vi "FGV Datenmanagment.vi"(11 "error in (no error)":errorcluster caption="Fehler (Eingang, kein Fehler)", 13 "Aktion":T3=enum."lesen") -> (2 "Aktuelle Messwerte":sgl[](array[numeric]), 3 "Ergebnistabelle":string[][](array[string]), 4 "Daten":T1 {"Höchster Peak" format="%#_5g"; "T10 Grenzwert" format="%#_5g"; "FallTime gemittelt" format="%#_5g"; "T90 Grenzwert" format="%#_5g"; "RiseTime gemittelt" format="%#_5g"}, 6 "T90 Signalverlauf":waveform(sgl) caption="Waveform", 8 "Peak im Bereich":bool, 10 "Aktueller Wert":sgl, 14 "Start":timestamp, 15 "error out":errorcluster caption="Fehler (Ausgang)")   [LabVIEW 2020, in "EPA 1065.lvlib" / "T90 Test 1065-308.lvlib"]
uses:
  T90 Test 1065-308.lvlib
  Aktion FGV Datenmanagment.ctl
  Datencluster.ctl
  Visualisierungs Elemente/Zahlen-Eingabefeld.ctl
  Aktion FGV T90.ctl
  Messdaten/Aktionen FGV Messdaten.ctl
  <vilib>/Analysis/baseanly.llb/Mean (DBL).vi
  Messdaten/Messdaten.lvlib
  <vilib>/Analysis/NI_AALBase.lvlib
panel:
  out "Umschaltzeitpunkt":timestamp[](array[timestamp])
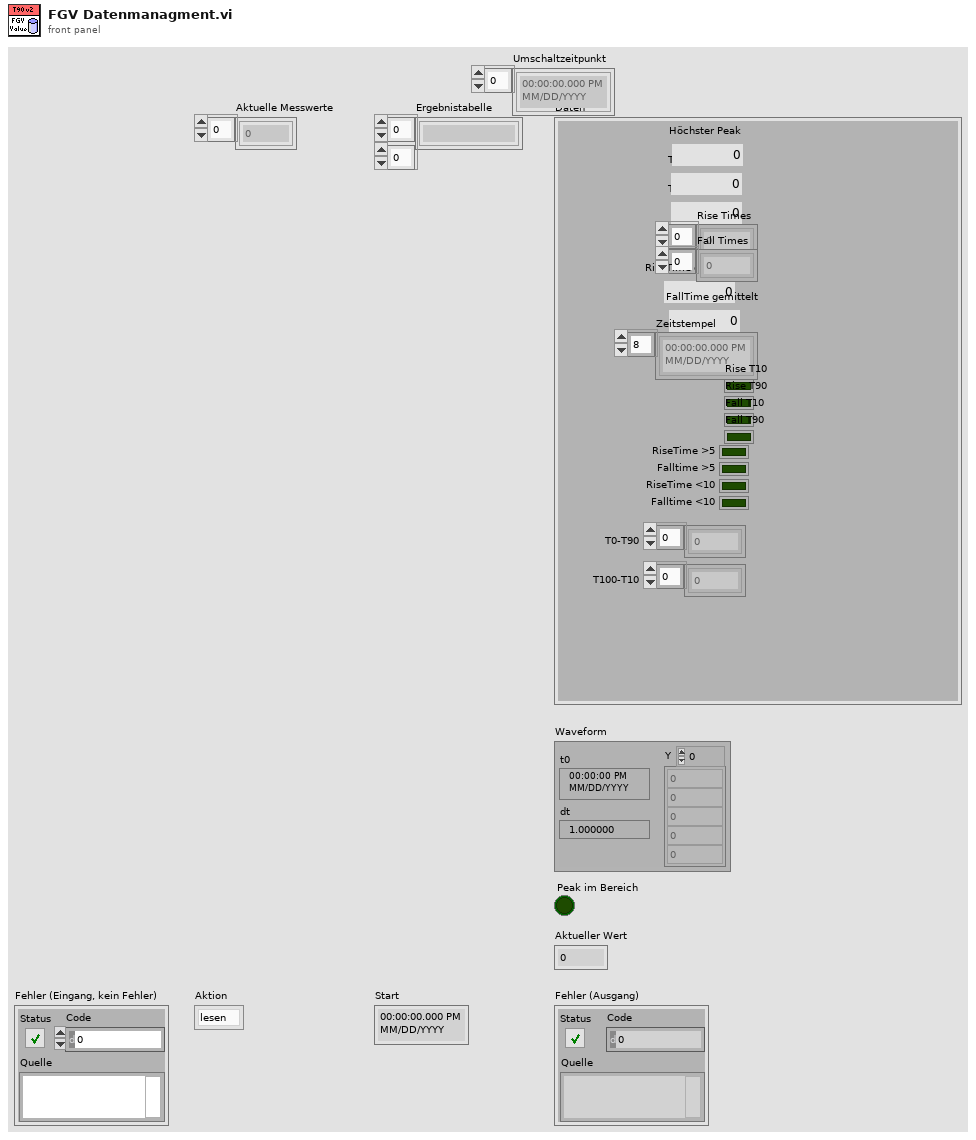
[diagram p1: front panel]
types:
  T1 = typedef "EPA 1065.lvlib/T90 Test 1065-308.lvlib/Datencluster.ctl" = cluster{"Höchster Peak":T2, "T10 Grenzwert":T2, "T90 Grenzwert":T2, "Rise Times":dbl[], "Fall Times":dbl[], "RiseTime gemittelt":T2, "FallTime gemittelt":T2, "Zeitstempel":timestamp[], "Rise T10":bool, "Rise T90":bool, "Fall T10":bool, "Fall T90":bool, "RiseTime >5":bool, "Falltime >5":bool, "RiseTime <10":bool, "Falltime <10":bool, "T0-T90":dbl[], "T100-T10":dbl[]}
  T2 = typedef "Zahlen-Eingabefeld.ctl" = sgl
  T3 = typedef "EPA 1065.lvlib/T90 Test 1065-308.lvlib/Aktion FGV Datenmanagment.ctl" = enum16{"init", "lesen", "Istwerte schreiben", "höchsten Peak setzen", "Auswerten", "Grenzen setzen", "Sollwert ändern", "Rise T10", "Rise T90", "Fall T90", "Fall T10", "Bit löschen", "Umschaltzeitpunkt"}
  T4 = typedef "EPA 1065.lvlib/T90 Test 1065-308.lvlib/Aktion FGV T90.ctl" = enum16{"lesen", "Konfig Daten", "speichern", "laden", "T90 aktiv", "T90 inaktiv", "Ext. Ventil aktivieren", "Ext. Ventil deaktivieren", "N2 spülen aktiv", "N2 spülen inaktiv", "Ergebnis Textfile"}
  T5 = typedef "Messdaten.lvlib/Aktionen FGV Messdaten.ctl" = enum16{"lesen", "schreiben", "löschen", "Mittelwerte", "Komponente"}
  T6 = typedef "EPA 1065.lvlib/T90 Test 1065-308.lvlib/T90 Konfig Daten.ctl" = cluster{"Bearbeiter:":string, "Komponente:":u16, "Gasflaschen Nr.:":string, "Accuracy":dbl, "Sollwert":dbl, "Modus":T7, "Abschaltzeit:":dbl, "Abweichung:":dbl, "Pfad:":path, "Textname:":string, "CG Aufschaltzeit:":dbl, "Einheit":string, "N2 Aufschaltzeit:":dbl, "Analysator":T8, "Gasflasche":T9, "Konfig Gasflasche":T10, "Frequency:":T11}
  T7 = typedef "EPA 1065.lvlib/T90 Test 1065-308.lvlib/Modus.ctl" = u16
  T8 = typedef "System Einstellungen V2.lvlib/Analysatoren.ctl" = string
  T9 = typedef "System Einstellungen V2.lvlib/Gasflasche Auswahl.ctl" = u16
  T10 = typedef "System Einstellungen V2.lvlib/Konfig Gasflasche.ctl" = bool
  T11 = typedef "EPA 1065.lvlib/T90 Test 1065-308.lvlib/Frequenz.ctl" = u16
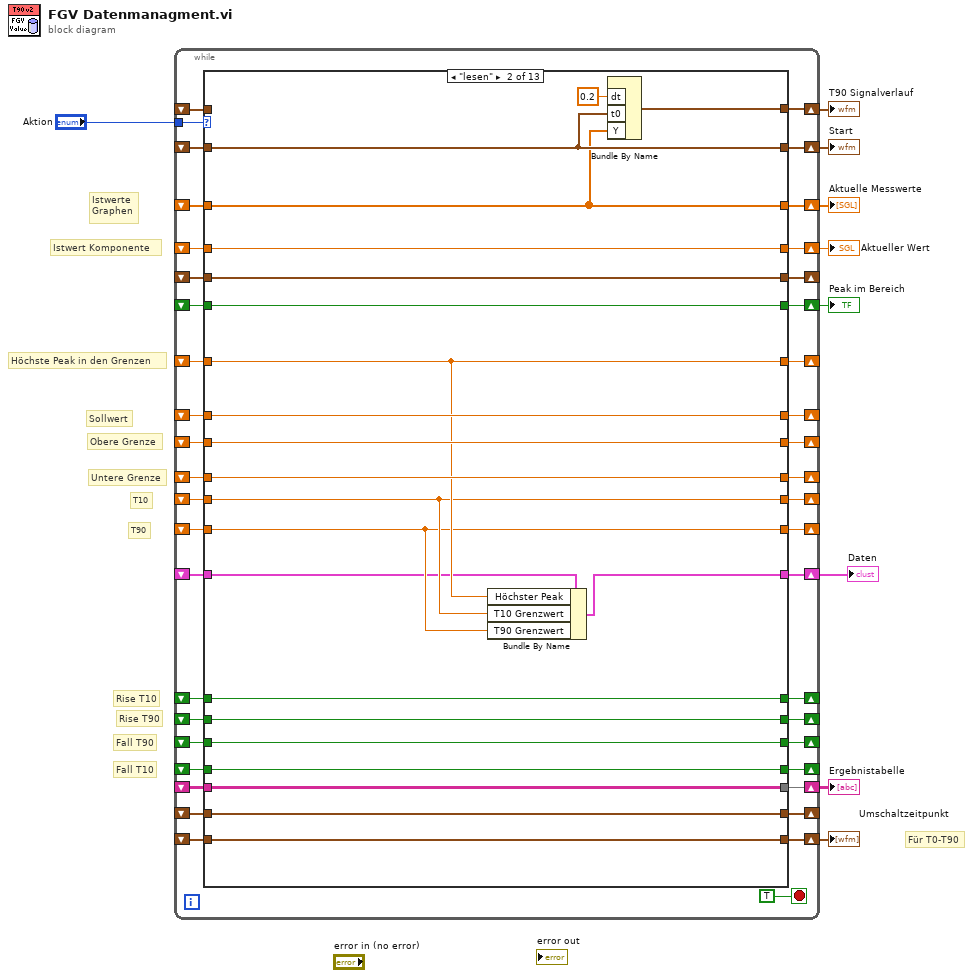
[diagram p0: block diagram]
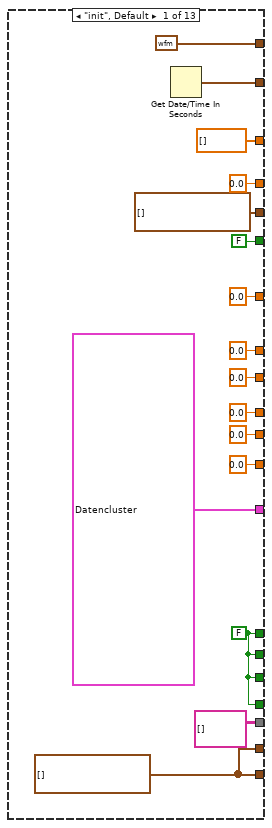
[diagram p2: hidden frame]
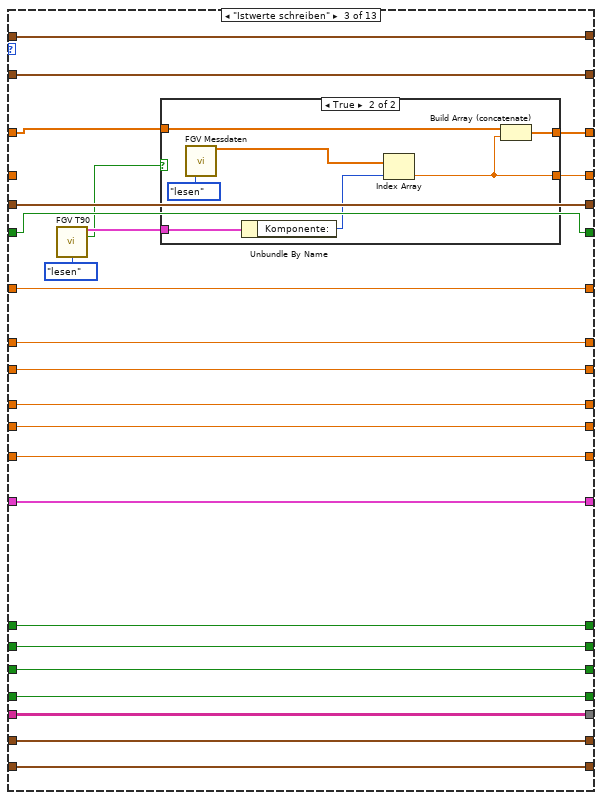
[diagram p3: hidden frame]
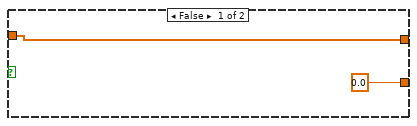
[diagram p4: hidden frame]
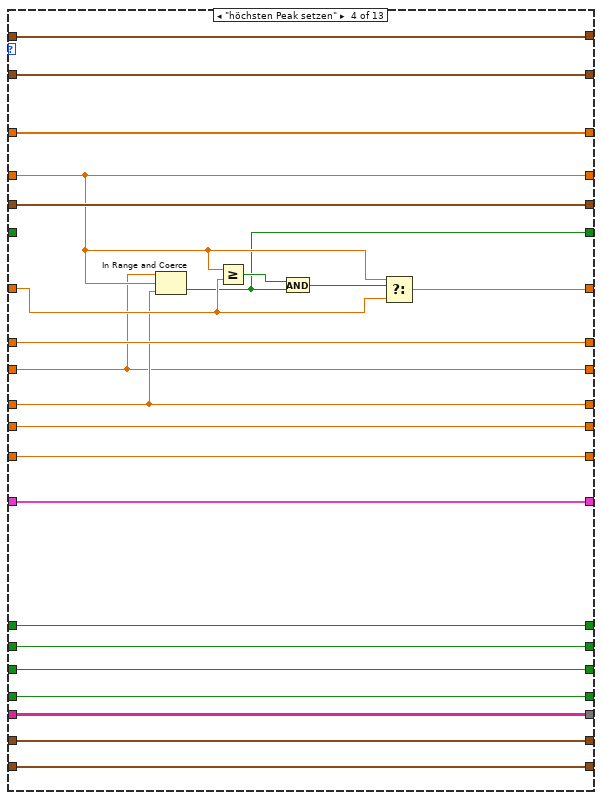
[diagram p5: hidden frame]
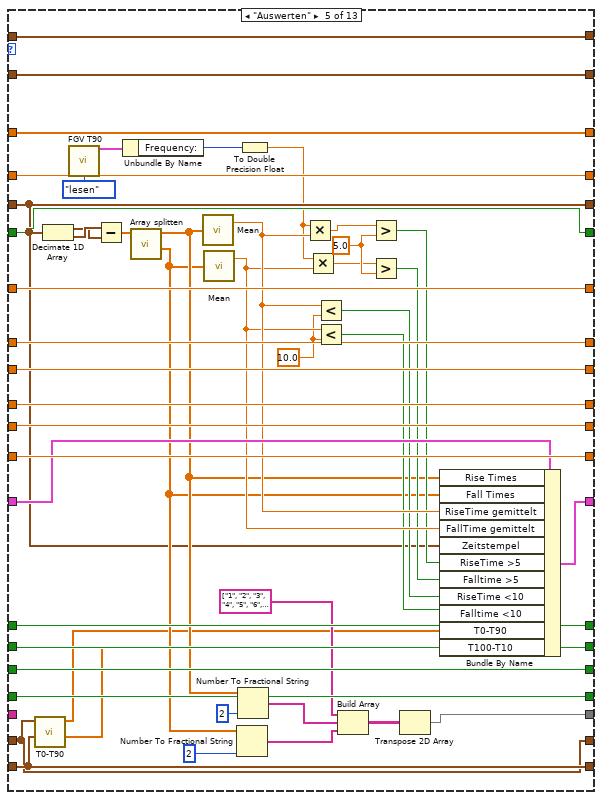
[diagram p6: hidden frame]
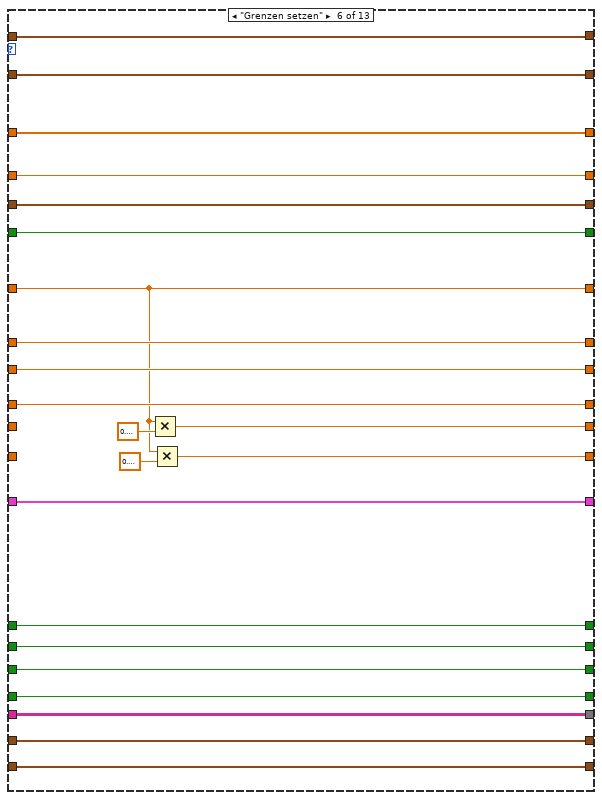
[diagram p7: hidden frame]
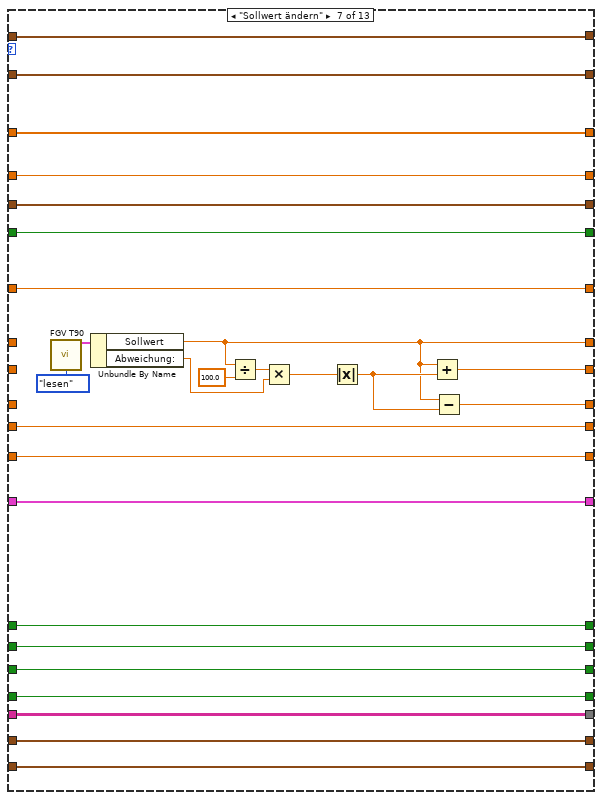
[diagram p8: hidden frame]
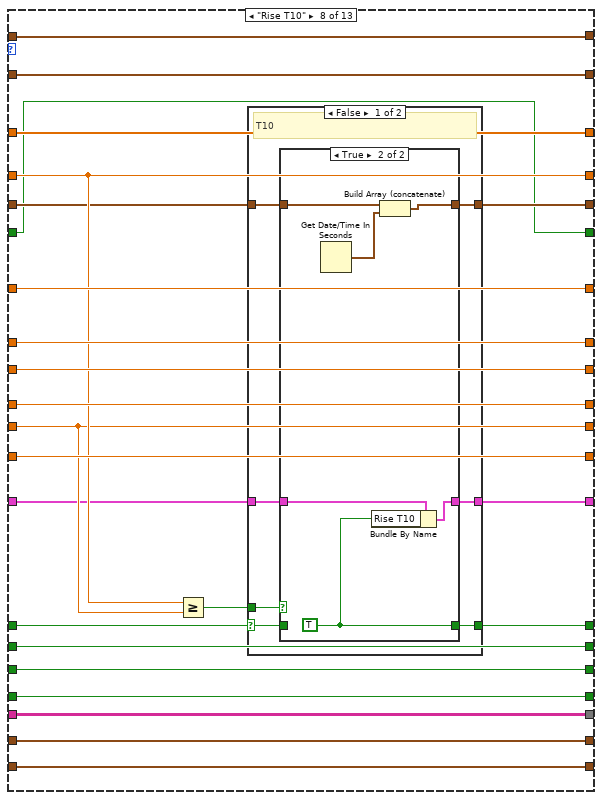
[diagram p9: hidden frame]
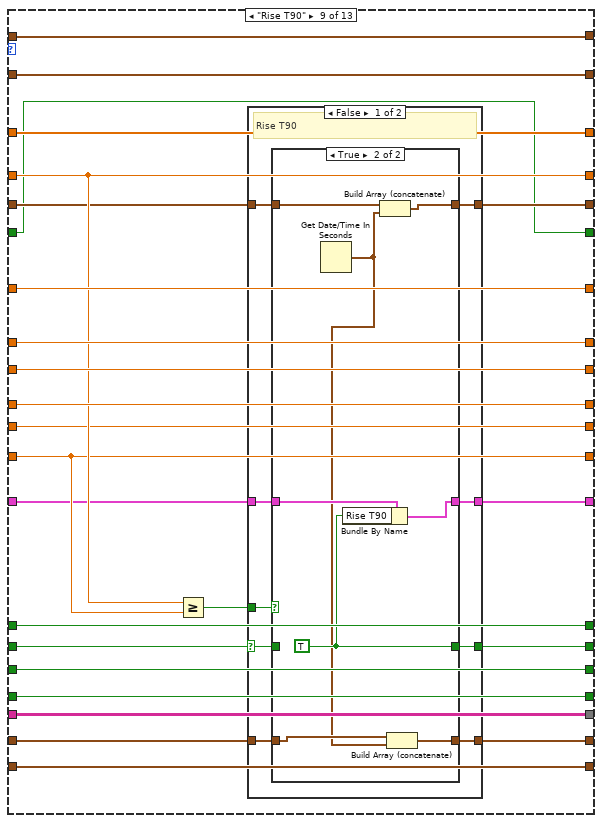
[diagram p12: hidden frame]
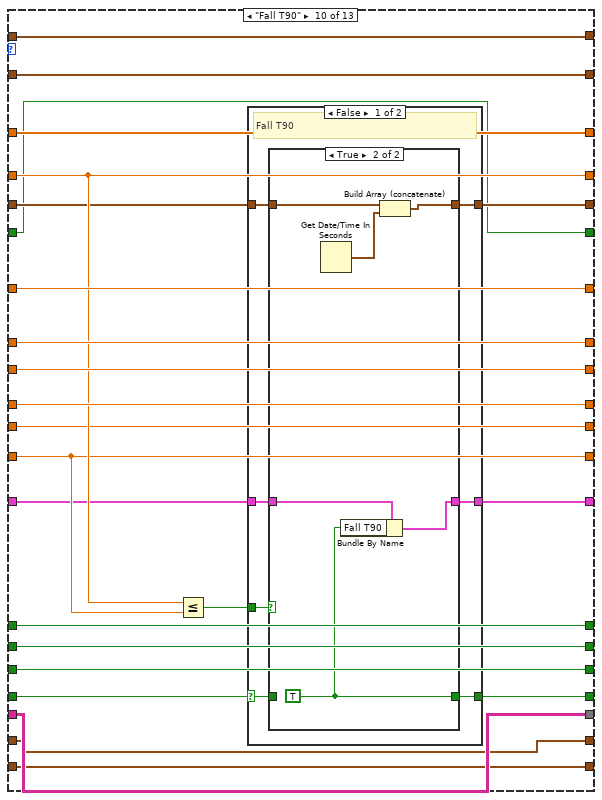
[diagram p15: hidden frame]
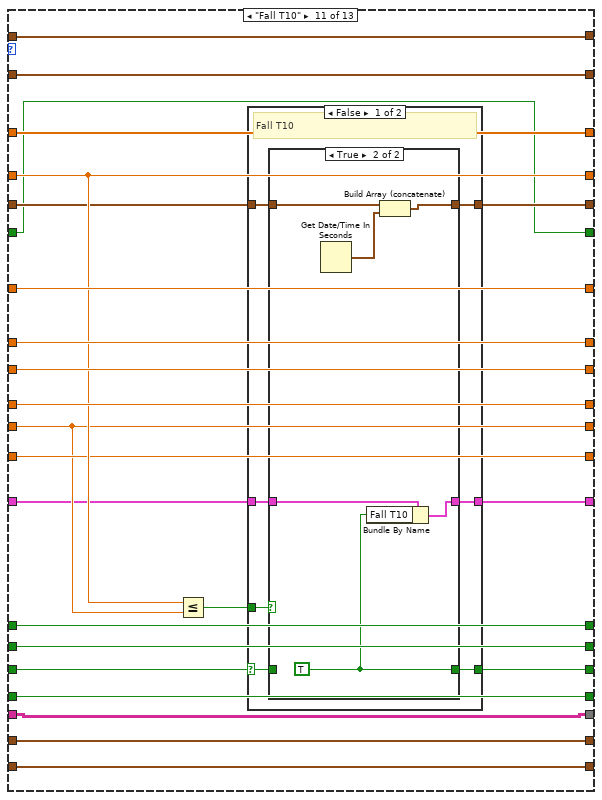
[diagram p18: hidden frame]
diagram:
  # "Für T0-T90"
  # "Fall T10"
  # "Fall T90"
  # "Rise T90"
  # "Rise T10"
  # "T90"
  # "T10"
  # "Untere Grenze"
  # "Obere Grenze"
  # "Sollwert"
  # "Höchste Peak in den Grenzen"
  # "Istwert Komponente"
  # "Istwerte\nGraphen"
  n1 = while {
    tunnel: "Aktion" -> [w50]
    shift-right: [w49] -> w1
    shift-left: _ -> [w48]
    shift-right: [w47] -> _
    shift-left: _ -> [w46]
    shift-right: [w45] -> w8
    shift-left: _ -> [w44]
    shift-right: [w43] -> _
    shift-left: _ -> [w42]
    shift-right: [w39] -> _
    shift-left: _ -> [w38]
    shift-right: [w41] -> _
    shift-left: _ -> [w37]
    shift-right: [w40] -> _
    shift-left: _ -> [w36]
    shift-right: [w35] -> _
    shift-left: _ -> [w34]
    shift-right: [w33] -> _
    shift-left: _ -> [w32]
    shift-right: [w31] -> w7
    shift-left: _ -> [w30]
    shift-right: [w28] -> _
    shift-left: _ -> [w27]
    shift-right: [w25] -> _
    shift-left: _ -> [w26]
    shift-right: [w23] -> _
    shift-left: _ -> [w24]
    shift-right: [w21] -> _
    shift-left: _ -> [w22]
    shift-right: [w20] -> w3
    shift-left: _ -> [w19]
    shift-right: [w18] -> w5
    shift-left: _ -> [w17]
    shift-right: [w16] -> w4
    shift-left: _ -> [w15]
    shift-right: [w29] -> w6
    shift-left: _ -> [w14]
    shift-right: [w13] -> w2
    shift-left: _ -> [w12]
    shift-right: [w11] -> _
    shift-left: _ -> [w10]
    stop <- TRUE stop-if-true
    n2 = case shown="\"lesen\"" w50 {
      tunnel: [sgl[] [] ("Aktuelle Messwerte") w74 w101 w145 w193 w215 w236 w266 w310 w359 w402 w436 w452] -> w49
      tunnel: w48 -> [_ w74 w100 w145 w193 w215 w236 w266 w310 w359 w402 w436 w452]
      tunnel: [timestamp[] [] w89 w113 w144 w154 w213 w234 w254 w301 w350 w394 w434 w450] -> w47
      tunnel: w46 -> [_ w89 w113 w144 w154 w213 w234 w255 w302 w351 w395 w434 w450]
      tunnel: [sgl 0.0 ("Numerisch") w88 w102 w139 w192 w214 w235 w258 w305 w354 w397 w435 w451] -> w45
      tunnel: w44 -> [_ w88 _ w139 w192 w214 w235 w258 w305 w354 w397 w435 w451]
      tunnel: [sgl 0.0 ("Numerisch") w84 w112 w141 w191 w197 w233 w265 w309 w358 w401 w433 w449] -> w43
      tunnel: w42 -> [_ w84 w112 w140 w191 w197 w233 w265 w309 w358 w401 w433 w449]
      tunnel: [T2 0.0 ("Sollwert") w87 w110 w126 w189 w212 w238 w263 w307 w356 w399 w431 w447] -> w41
      tunnel: [T2 0.0 ("Sollwert") w85 w111 w138 w190 w207 w223 w264 w308 w357 w400 w432 w448] -> w40
      tunnel: [T2 0.0 ("Sollwert") w86 w109 w137 w188 w211 w237 w262 w306 w355 w398 w430 w446] -> w39
      tunnel: w38 -> [_ w86 w109 w137 w188 w211 _ w262 w306 w355 w398 w430 w446]
      tunnel: w37 -> [_ w87 w110 w126 w189 w212 _ w263 w307 w356 w399 w431 w447]
      tunnel: w36 -> [_ w85 w111 w138 w190 w207 _ w264 w308 w357 w400 w432 w448]
      tunnel: [T2 0.0 ("Sollwert") w83 w108 w136 w187 w209 w232 w257 w304 w353 w388 w429 w445] -> w35
      tunnel: w34 -> [_ w83 w108 w136 w187 _ w232 w257 w304 w353 w388 w429 w445]
      tunnel: [T2 0.0 ("Sollwert") w82 w107 w135 w186 w206 w231 w261 w300 w349 w393 w428 w444] -> w33
      tunnel: w32 -> [_ w82 w107 w135 w186 _ w231 w261 w300 w349 w393 w428 w444]
      tunnel: [T1 {"Höchster Peak"=0.0, "T10 Grenzwert"=0.0, "T90 Grenzwert"=0.0, "Rise Times"=[0.0, 0.0, 0.0, 0.0, 0.0, 0.0, 0.0, 0.0, 0.0, 0.0, 0.0], "Fall Times"=[0.0, 0.0, 0.0, 0.0, 0.0, 0.0, 0.0, 0.0, 0.0, 0.0, 0.0], "RiseTime gemittelt"=0.0, "FallTime gemittelt"=0.0, "Zeitstempel"=[timestamp(0 s since 1904-01-01), timestamp(0 s since 1904-01-01), timestamp(0 s since 1904-01-01), timestamp(0 s since 1904-01-01), timestamp(0 s since 1904-01-01), timestamp(0 s since 1904-01-01), timestamp(0 s since 1904-01-01), timestamp(0 s since 1904-01-01), timestamp(0 s since 1904-01-01), timestamp(0 s since 1904-01-01), timestamp(0 s since 1904-01-01), timestamp(0 s since 1904-01-01), timestamp(0 s since 1904-01-01), timestamp(0 s since 1904-01-01), timestamp(0 s since 1904-01-01), timestamp(0 s since 1904-01-01), timestamp(0 s since 1904-01-01), timestamp(0 s since 1904-01-01), timestamp(0 s since 1904-01-01), timestamp(0 s since 1904-01-01), timestamp(0 s since 1904-01-01), timestamp(0 s since 1904-01-01), timestamp(0 s since 1904-01-01), timestamp(0 s since 1904-01-01), timestamp(0 s since 1904-01-01), timestamp(0 s since 1904-01-01), timestamp(0 s since 1904-01-01), timestamp(0 s since 1904-01-01), timestamp(0 s since 1904-01-01), timestamp(0 s since 1904-01-01), timestamp(0 s since 1904-01-01), timestamp(0 s since 1904-01-01), timestamp(0 s since 1904-01-01), timestamp(0 s since 1904-01-01), timestamp(0 s since 1904-01-01), timestamp(0 s since 1904-01-01), timestamp(0 s since 1904-01-01), timestamp(0 s since 1904-01-01), timestamp(0 s since 1904-01-01), timestamp(0 s since 1904-01-01), timestamp(0 s since 1904-01-01), timestamp(0 s since 1904-01-01), timestamp(0 s since 1904-01-01), timestamp(0 s since 1904-01-01), timestamp(0 s since 1904-01-01), timestamp(0 s since 1904-01-01), timestamp(0 s since 1904-01-01), timestamp(0 s since 1904-01-01), timestamp(0 s since 1904-01-01), timestamp(0 s since 1904-01-01), timestamp(-3600 s since 1904-01-01)], "Rise T10"=FALSE, "Rise T90"=FALSE, "Fall T10"=FALSE, "Fall T90"=FALSE, "RiseTime >5"=FALSE, "Falltime >5"=FALSE, "RiseTime <10"=FALSE, "Falltime <10"=FALSE, "T0-T90"=[], "T100-T10"=[]} ("Daten") w81 w96 w134 w184 w205 w230 w249 w293 w342 w385 w438 w461] -> w31
      tunnel: w30 -> [_ w80 w96 w134 w185 w205 w230 w250 w294 w343 w386 w439 w461]
      tunnel: [FALSE w70 w93 w125 w161 w196 w218 w245 w289 w338 w381 w424 w460] -> w29
      tunnel: [w58 w79 w106 w133 w183 w204 w229 w260 w297 w348 w390 w437 w459] -> w28
      tunnel: w27 -> [_ w79 w106 w133 w183 w204 w229 w259 w297 w348 w390 _ w459]
      tunnel: w26 -> [_ w78 w105 w132 w182 w203 w228 w253 w298 w347 w389 _ w458]
      tunnel: [w58 w78 w105 w132 w182 w203 w228 w253 w299 w347 w389 w437 w458] -> w25
      tunnel: w24 -> [_ w77 w104 w131 w181 w202 w227 w252 w296 w344 w391 _ w457]
      tunnel: [w58 w77 w104 w131 w181 w202 w227 w252 w296 w344 w392 w437 w457] -> w23
      tunnel: w22 -> [_ w76 w103 w130 w180 w201 w226 w251 w295 w345 w387 _ w456]
      tunnel: [w58 w76 w103 w130 w180 w201 w226 w251 w295 w346 w387 w437 w456] -> w21
      tunnel: [w57 w75 w99 w129 w179 w200 w221 w248 w292 w341 w384 w427 w455] -> w20
      tunnel: w19 -> [_ w75 w99 w129 w179 w200 w221 w248 w292 w341 w384 w427 w455]
      tunnel: [waveform(sgl) {"t0"=timestamp(0 s since 1904-01-01), "dt"=1.0, "Y"=[]} w72 w98 w128 w178 w199 w220 w247 w291 w340 w383 w426 w454] -> w18
      tunnel: w17 -> [_ _ w98 w128 w178 w199 w220 w247 w291 w340 w383 w426 w454]
      tunnel: [string[][] [] w71 w97 w127 w156 w198 w219 w246 w290 w339 w382 w425 w453] -> w16
      tunnel: w15 -> [_ w71 w97 w127 _ w198 w219 w246 w290 w339 w382 w425 w453]
      tunnel: w14 -> [_ w70 w93 _ w161 w196 w218 w245 w289 w338 w381 w424 w460]
      tunnel: [w52 w69 w91 w124 w155 w195 w217 w244 w288 w337 w380 w423 w443] -> w13
      tunnel: w12 -> [_ w69 w91 w124 w155 w195 w217 w244 w288 w337 w380 w423 w441]
      tunnel: [w52 w68 w90 w123 w150 w194 w216 w243 w287 w336 w379 w422 w440] -> w11
      tunnel: w10 -> [_ w68 w90 w123 w150 w194 w216 w243 w286 w336 w379 w422 w440]
      frame "init", Default {
        w52 = timestamp[] [] ("Umschaltzeitpunkt")
        w58 = FALSE
        n3 = Get Date/Time In Seconds() -> (seconds since 1Jan1904=w57:timestamp)
      }
      frame "lesen" {
        n4 = Bundle By Name(cluster=w80, "Höchster Peak"=w84, "T10 Grenzwert"=w83, "T90 Grenzwert"=w82) -> (w81:T1)
        n5 = Bundle By Name("dt"=0.2, "t0"=w75, "Y"=w74) -> (w72:waveform(sgl))  [unwired: 1 in]
      }
      frame "Istwerte schreiben" {
        n6 = call "FGV T90.vi"("Aktion"=Aktion_FGV_T90."lesen") -> ("T90 Konfig Daten"=w94:T6, "T90 Aktiv"=w92:bool)  [unwired: 9 in, 4 out]
        n7 = case shown="True" w92 {
          tunnel: [sgl 0.0 ("Numerisch") w120] -> w102
          tunnel: [w114 w119] -> w101
          tunnel: w100 -> [w114 w118]
          tunnel: w94 -> [_ w117]
          frame False {
          }
          frame True {
            n8 = call "FGV Messdaten.vi"("Aktionen"=Aktionen_FGV_Messdaten."lesen") -> ("Aktuelle Messwerte"=w121:sgl[])  [unwired: 6 in, 8 out]
            n9 = Unbundle By Name(w117) -> ("Komponente:"=w116:u16)
            n10 = Index Array(array=w121, index=w116) -> (element=w120:sgl)
            n11 = Build Array (concatenate)(w118, w120) -> (w119:sgl[])
          }
        }
      }
      frame "höchsten Peak setzen" {
        n12 = In Range and Coerce(upper limit=w126, x=w139, lower limit=w137) -> (In Range?=w125:bool)  [unwired: 1 out]
        n13 = Greater Or Equal?(x=w139, y=w140) -> (x >= y?=w142:bool)
        n14 = And(x=w142, y=w125) -> (x .and. y?=w143:bool)
        n15 = Select(t=w139, s=w143, f=w140) -> (s? t:f=w141:sgl)
      }
      frame "Auswerten" {
        w172 = 10.0 ("y")
        w176 = 5.0 ("Hz")
        n16 = call "T0-T90.vi"("Umschaltzeitpunkte"=w155, "T0-T90"=w150) -> ("T100-T10"=w152:dbl[], "T0-T90"=w153:dbl[])  [unwired: 7 in, 1 out]
        n17 = Decimate 1D Array(w154) -> (w159:timestamp[], w160:timestamp[])
        n18 = call "FGV T90.vi"("Aktion"=Aktion_FGV_T90."lesen") -> ("T90 Konfig Daten"=w148:T6)  [unwired: 9 in, 5 out]
        n19 = Subtract(x=w160, y=w159) -> (x-y=w151:dbl[])
        n20 = Unbundle By Name(w148) -> ("Frequency:"=w147:T11)
        n21 = call "Array splitten.vi"("Array"=w151) -> ("Ungerader Index"=w157:dbl[], "Gerader Index"=w158:dbl[])  [unwired: 8 in, 1 out]
        n22 = call-poly <vilib>:"Mean.vi"("X"=w158) -> ("mean"=w174:dbl)  [unwired: 1 out]
        n23 = call-poly <vilib>:"Mean.vi"("X"=w157) -> ("mean"=w173:dbl)  [unwired: 1 out]
        n24 = Number To Fractional String(number=w157, precision (6)=i16 2 ("Genauigkeit (6)")) -> (F-format string=w163:string[])  [unwired: 2 in]
        n25 = Number To Fractional String(number=w158, precision (6)=i16 2 ("Genauigkeit (6)")) -> (F-format string=w164:string[])  [unwired: 2 in]
        n26 = To Double Precision Float(number=w147) -> (double precision float=w146:dbl)
        n27 = Multiply(x=w146, y=w174) -> (x*y=w177:dbl)
        n28 = Multiply(x=w146, y=w173) -> (x*y=w175:dbl)
        n29 = Less?(x=w174, y=w172) -> (x < y?=w170:bool)
        n30 = Less?(x=w173, y=w172) -> (x < y?=w168:bool)
        n31 = Build Array(string[] ["1", "2", "3", "4", "5", "6", "7"], w164, w163) -> (w162:string[][])
        n32 = Greater?(x=w177, y=w176) -> (0:w171:bool)
        n33 = Greater?(x=w175, y=w176) -> (0:w169:bool)
        n34 = Transpose 2D Array(2D array=w162) -> (transposed array=w156:string[][])
        n35 = Bundle By Name(cluster=w185, "Rise Times"=w158, "Fall Times"=w157, "RiseTime gemittelt"=w174, "FallTime gemittelt"=w173, "Zeitstempel"=w154, "RiseTime >5"=w171, "Falltime >5"=w169, "RiseTime <10"=w170, "Falltime <10"=w168, "T0-T90"=w153, "T100-T10"=w152) -> (w184:T1)
      }
      frame "Grenzen setzen" {
        n36 = Multiply(x=w197, y=T2 0.1) -> (x*y=w209:T2)
        n37 = Multiply(x=w197, y=T2 0.9) -> (x*y=w206:T2)
      }
      frame "Sollwert ändern" {
        n38 = call "FGV T90.vi"("Aktion"=Aktion_FGV_T90."lesen") -> ("T90 Konfig Daten"=w224:T6)  [unwired: 9 in, 5 out]
        n39 = Unbundle By Name(w224) -> ("Sollwert"=w223:dbl, "Abweichung:"=w222:dbl)
        n40 = Divide(x=w223, y=T2 100.0) -> (x/y=w242:dbl)
        n41 = Multiply(x=w242, y=w222) -> (x*y=w241:dbl)
        n42 = Absolute Value(x=w241) -> (abs(x)=w239:dbl)
        n43 = Add(x=w223, y=w239) -> (x+y=w238:dbl)
        n44 = Subtract(x=w223, y=w239) -> (x-y=w237:dbl)
      }
      frame "Rise T10" {
        n45 = Greater Or Equal?(x=w258, y=w257) -> (x >= y?=w256:bool)
        n46 = case shown="False" w259 {
          selector: w259 -> [w271 w285]
          tunnel: [w273 w285] -> w260
          tunnel: w256 -> [w272 _]
          tunnel: w255 -> [w270 w284]
          tunnel: [w269 w284] -> w254
          tunnel: w250 -> [w268 w283]
          tunnel: [w267 w283] -> w249
          frame False {
            # "T10"
            n47 = case shown="True" w272 {
              tunnel: [w276 w277] -> w273
              tunnel: w271 -> [w276 _]
              tunnel: w270 -> [w275 w282]
              tunnel: [w275 w280] -> w269
              tunnel: w268 -> [w274 w279]
              tunnel: [w274 w278] -> w267
              frame False {
              }
              frame True {
                w277 = TRUE
                n48 = Get Date/Time In Seconds() -> (seconds since 1Jan1904=w281:timestamp)
                n49 = Bundle By Name(cluster=w279, "Rise T10"=w277) -> (w278:T1)
                n50 = Build Array (concatenate)(w282, w281) -> (w280:timestamp[])
              }
            }
          }
          frame True {
          }
        }
      }
      frame "Rise T90" {
        n51 = Greater Or Equal?(x=w305, y=w300) -> (x >= y?=w303:bool)
        n52 = case shown="False" w298 {
          selector: w298 -> [w317 w335]
          tunnel: [w319 w335] -> w299
          tunnel: w303 -> [w318 _]
          tunnel: w302 -> [w316 w334]
          tunnel: [w315 w334] -> w301
          tunnel: w294 -> [w314 w333]
          tunnel: [w313 w333] -> w293
          tunnel: [w312 w332] -> w287
          tunnel: w286 -> [w311 w332]
          frame False {
            # "Rise T90"
            n53 = case shown="True" w318 {
              tunnel: [w323 w327] -> w319
              tunnel: w317 -> [w323 _]
              tunnel: w316 -> [w322 w331]
              tunnel: [w322 w330] -> w315
              tunnel: w314 -> [w321 w329]
              tunnel: [w321 w328] -> w313
              tunnel: [w320 w326] -> w312
              tunnel: w311 -> [w320 w325]
              frame False {
              }
              frame True {
                w327 = TRUE
                n54 = Get Date/Time In Seconds() -> (seconds since 1Jan1904=w324:timestamp)
                n55 = Bundle By Name(cluster=w329, "Rise T90"=w327) -> (w328:T1)
                n56 = Build Array (concatenate)(w331, w324) -> (w330:timestamp[])
                n57 = Build Array (concatenate)(w325, w324) -> (w326:timestamp[])
              }
            }
          }
          frame True {
          }
        }
      }
      frame "Fall T90" {
        n58 = Less Or Equal?(x=w354, y=w349) -> (x <= y?=w352:bool)
        n59 = case shown="False" w345 {
          selector: w345 -> [w364 w378]
          tunnel: [w366 w378] -> w346
          tunnel: w352 -> [w365 _]
          tunnel: w351 -> [w363 w377]
          tunnel: [w362 w377] -> w350
          tunnel: w343 -> [w361 w376]
          tunnel: [w360 w376] -> w342
          frame False {
            # "Fall T90"
            n60 = case shown="True" w365 {
              tunnel: [w369 w370] -> w366
              tunnel: w364 -> [w369 _]
              tunnel: w363 -> [w368 w375]
              tunnel: [w368 w373] -> w362
              tunnel: w361 -> [w367 w372]
              tunnel: [w367 w371] -> w360
              frame False {
              }
              frame True {
                w370 = TRUE
                n61 = Get Date/Time In Seconds() -> (seconds since 1Jan1904=w374:timestamp)
                n62 = Bundle By Name(cluster=w372, "Fall T90"=w370) -> (w371:T1)
                n63 = Build Array (concatenate)(w375, w374) -> (w373:timestamp[])
              }
            }
          }
          frame True {
          }
        }
      }
      frame "Fall T10" {
        n64 = Less Or Equal?(x=w397, y=w388) -> (x <= y?=w396:bool)
        n65 = case shown="False" w391 {
          selector: w391 -> [w407 w421]
          tunnel: [w409 w421] -> w392
          tunnel: w396 -> [w408 _]
          tunnel: w395 -> [w406 w420]
          tunnel: [w405 w420] -> w394
          tunnel: w386 -> [w404 w419]
          tunnel: [w403 w419] -> w385
          frame False {
            # "Fall T10"
            n66 = case shown="True" w408 {
              tunnel: [w412 w413] -> w409
              tunnel: w407 -> [w412 _]
              tunnel: w406 -> [w411 w418]
              tunnel: [w411 w416] -> w405
              tunnel: w404 -> [w410 w415]
              tunnel: [w410 w414] -> w403
              frame False {
              }
              frame True {
                w413 = TRUE
                n67 = Get Date/Time In Seconds() -> (seconds since 1Jan1904=w417:timestamp)
                n68 = Bundle By Name(cluster=w415, "Fall T10"=w413) -> (w414:T1)
                n69 = Build Array (concatenate)(w418, w417) -> (w416:timestamp[])
              }
            }
          }
          frame True {
          }
        }
      }
      frame "Bit löschen" {
        w437 = FALSE
        n70 = Bundle By Name(cluster=w439, "Rise T10"=w437, "Rise T90"=w437, "Fall T10"=w437, "Fall T90"=w437) -> (w438:T1)
      }
      frame "Umschaltzeitpunkt" {
        n71 = Get Date/Time In Seconds() -> (seconds since 1Jan1904=w442:timestamp)
        n72 = Build Array (concatenate)(w441, w442) -> (w443:timestamp[])
      }
    }
  }
  "Aktueller Wert" <- w8
  "Daten" <- w7
  "Peak im Bereich" <- w6
  "T90 Signalverlauf" <- w5
  "Ergebnistabelle" <- w4
  "Start" <- w3
  "Umschaltzeitpunkt" <- w2
  "Aktuelle Messwerte" <- w1
